vi "bubbles.vi"(4 "Direction":bool, 5 "in":dbl[](array[numeric])) -> (0 "out":dbl[](array[numeric]))   [LabVIEW 2024]
panel:
  # "ASC"
  # "DESC"
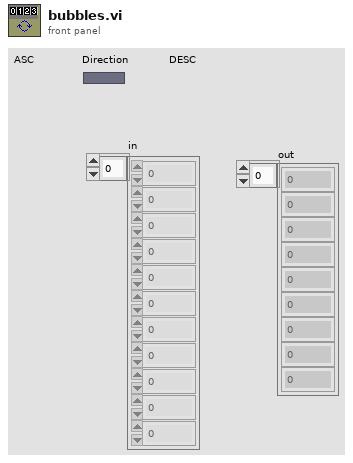
[diagram p1: front panel]
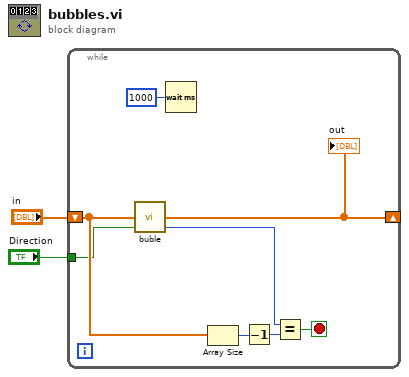
[diagram p0: block diagram]
diagram:
  n1 = while {
    shift-right: [w8] -> _
    shift-left: "in" -> [w10]
    tunnel: "Direction" -> [w3]
    stop <- w9 stop-if-true
    n2 = call "buble.vi"("Direction"=w3, "in"=w10) -> ("counter"=w7:i32, "out"=w8:dbl[])  [unwired: 2 in]
    "out" <- w8
    n3 = Wait (ms)(milliseconds to wait=u32 1000) -> ()  [unwired: 1 out]
    n4 = Array Size(array=w10) -> (size(s)=w6:i32)
    n5 = Decrement(x=w6) -> (x-1=w5:i32)
    n6 = Equal?(x=w7, y=w5) -> (x = y?=w9:bool)
  }
